vi "Write N LEDs.vi"(7 "Refresh? (T)":bool=TRUE, 8 "Error In":errorcluster, 9 "Colors":u32[](array[colorbox]), 10 "LED Index":u16, 11 "LINX Ref":T1={"IO"=enum."Remote", "Interface"=enum."Serial", "LINX Device Config"={"Interface"=enum."Serial", "COM Port"="COM13", "TCP Configuration"={"IP Address"="", "Port"=0}, "Device Family"=1, "Device ID"=1, "Device Name"="myRIO-1900", "TCP Ref"=refnum, "Channels"={"DI"=[0, 1, 2, 3, 4, 5, 6, 7, 8, 9, 10, 11, 12, 13, 14, 15, 16, 17, 18, 19, 20, 21, 22, 23, 24, 25, 26, 27, 28, 29, 30, 31, 32, 33, 34, 35, 36, 37, 38, 39, 40, 41, 42, 43, 44, 45, 46], "DO"=[0, 1, 2, 3, 4, 5, 6, 7, 8, 9, 10, 11, 12, 13, 14, 15, 16, 17, 18, 19, 20, 21, 22, 23, 24, 25, 26, 27, 28, 29, 30, 31, 32, 33, 34, 35, 36, 37, 38, 39, 40, 41, 42, 43, 44, 45, 46], "AI"=[0, 1, 2, 3, 4, 5, 6, 7, 8, 9, 10, 11], "AO"=[], "PWM"=[3, 5, 6, 9, 10], "QE"=[], "UART"=[0, 1], "I2C 2"=[0], "SPI"=[0], "CAN"=[], "Servo"=[], "AI Ref (V)"=0.0, "AI Resolution (Bits)"=0, "AO Ref (V)"=0.0, "AO Resolution (Bits)"=0}}}) -> (0 "Error Out":errorcluster, 3 "LINX Ref":T1={"IO"=enum."Remote", "Interface"=enum."Serial", "LINX Device Config"={"Interface"=enum."Serial", "COM Port"="COM13", "TCP Configuration"={"IP Address"="", "Port"=0}, "Device Family"=1, "Device ID"=1, "Device Name"="myRIO-1900", "TCP Ref"=refnum, "Channels"={"DI"=[0, 1, 2, 3, 4, 5, 6, 7, 8, 9, 10, 11, 12, 13, 14, 15, 16, 17, 18, 19, 20, 21, 22, 23, 24, 25, 26, 27, 28, 29, 30, 31, 32, 33, 34, 35, 36, 37, 38, 39, 40, 41, 42, 43, 44, 45, 46], "DO"=[0, 1, 2, 3, 4, 5, 6, 7, 8, 9, 10, 11, 12, 13, 14, 15, 16, 17, 18, 19, 20, 21, 22, 23, 24, 25, 26, 27, 28, 29, 30, 31, 32, 33, 34, 35, 36, 37, 38, 39, 40, 41, 42, 43, 44, 45, 46], "AI"=[0, 1, 2, 3, 4, 5, 6, 7, 8, 9, 10, 11], "AO"=[], "PWM"=[3, 5, 6, 9, 10], "QE"=[], "UART"=[0, 1], "I2C 2"=[0], "SPI"=[0], "CAN"=[], "Servo"=[], "AI Ref (V)"=0.0, "AI Resolution (Bits)"=0, "AO Ref (V)"=0.0, "AO Resolution (Bits)"=0}}})   [LabVIEW 2020, in "LMH-LINX.lvlib" / "WS2812.lvlib"]
doc: "Set the R, G, B color of N LEDs starting at the user specififed LED index. If Refresh is true (default) the new colors are immediatly displayed. If Refresh is false the new colors are stored in memory but the LEDs are not updated until Refresh is called."
uses:
  WS2812.lvlib
  Private/Type Defs/LINX Ref.ctl
  Private/Type Defs/Platform.ctl
  Private/Type Defs/Interface.ctl
  Private/Device/Type Defs/LINX Device Config.ctl
  Private/Device/Type Defs/TCP Config.ctl
  Private/Device/Type Defs/Channels.ctl
  Private/Type Defs/Error Type.ctl
  LMH-LINX.lvlib
  Private/Device/Device.lvlib
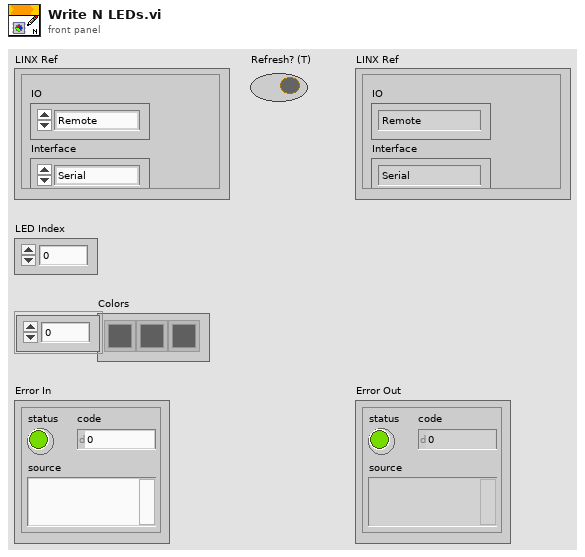
[diagram p1: front panel]
types:
  T1 = typedef "LMH-LINX.lvlib/LINX Ref.ctl" = cluster{"IO":T2, "Interface":T3, "LINX Device Config":T4}
  T2 = typedef "LMH-LINX.lvlib/Platform.ctl" = enum16{"Remote", "Local"}
  T3 = typedef "LMH-LINX.lvlib/Interface.ctl" = enum16{"Serial", "TCP"}
  T4 = typedef "Device.lvlib/LINX Device Config.ctl" = cluster{"Interface":T3, "COM Port":refnum<visa-resource-name>, "TCP Configuration":T5, "Device Family":u8, "Device ID":u8, "Device Name":string, "TCP Ref":refnum<k5>, "Channels":T6}
  T5 = typedef "Device.lvlib/TCP Config.ctl" = cluster{"IP Address":string, "Port":u16}
  T6 = typedef "LMH-LINX.lvlib/Channels.ctl" = cluster{"DI":u8[], "DO":u8[], "AI":u8[], "AO":u8[], "PWM":u8[], "QE":u8[], "UART":u8[], "I2C 2":u8[], "SPI":u8[], "CAN":u8[], "Servo":u8[], "AI Ref (V)":dbl, "AI Resolution (Bits)":u8, "AO Ref (V)":dbl, "AO Resolution (Bits)":u8}
  T7 = typedef "LMH-LINX.lvlib/Error Type.ctl" = enum16{"Unknown", "Timeout", "Corrupt Return Packet", "Unable To Connect", "Command Not Supported", "Channel DNE", "Invalid COM Config", "Firmware Version Mismatch", "myRIO Support", "CMD Specific Error", "Local IO Not Supported"}
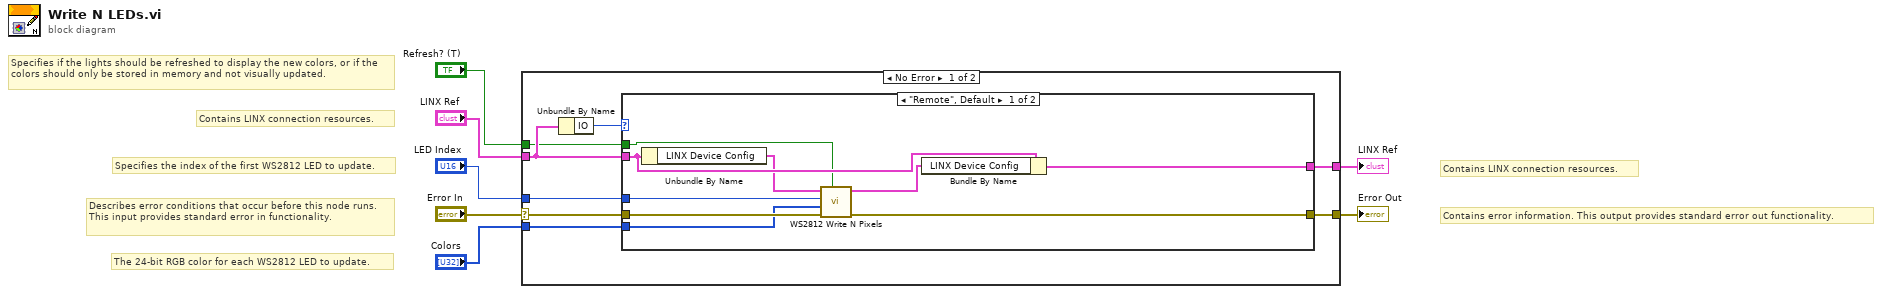
[diagram p0: block diagram]
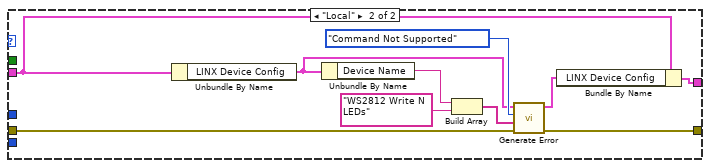
[diagram p2: hidden frame]
diagram:
  # "Specifies if the lights should be refreshed to display the new colors, or if the colors should only be stored in memory and not visually updated."
  # "Specifies the index of the first WS2812 LED to update."
  # "The 24-bit RGB color for each WS2812 LED to update."
  # "Contains LINX connection resources."
  # "Contains error information. This output provides standard error out functionality."
  # "Contains LINX connection resources."
  # "Describes error conditions that occur before this node runs. This input provides standard error in functionality."
  n1 = case shown="No Error" "Error In" {
    selector: "Error In" -> [w14 w35]
    tunnel: "LINX Ref" -> [w13 w36]
    tunnel: [w12 w35] -> w5
    tunnel: [w11 w36] -> w4
    tunnel: "LED Index" -> [w10 _]
    tunnel: "Colors" -> [w9 _]
    tunnel: "Refresh? (T)" -> [w8 _]
    frame No Error {
      n2 = Unbundle By Name(w13) -> ("IO"=w15:T2)
      n3 = case shown="\"Remote\", Default" w15 {
        tunnel: w14 -> [w21 w28]
        tunnel: w13 -> [w24 w25]
        tunnel: [w22 w27] -> w12
        tunnel: [w23 w26] -> w11
        tunnel: w10 -> [w17 _]
        tunnel: w9 -> [w16 _]
        tunnel: w8 -> [w18 _]
        frame "Remote", Default {
          n4 = Unbundle By Name(w24) -> ("LINX Device Config"=w20:T4)
          n5 = call "WS2812 Write N Pixels.vi"("Refresh?"=w18, "Error In"=w21, "Colors"=w16, "Start Pixel Index"=w17, "LINX Device Config"=w20) -> ("Error Out"=w22:errorcluster, "LINX Device Config"=w19:T4)  [unwired: 5 in]
          n6 = Bundle By Name(cluster=w24, "LINX Device Config"=w19) -> (w23:T1)
        }
        frame "Local" {
          n7 = Unbundle By Name(w25) -> ("LINX Device Config"=w30:T4)
          n8 = Unbundle By Name(w30) -> ("Device Name"=w34:string)
          n9 = Build Array(w34, "WS2812 Write N LEDs") -> (w31:string[])
          n10 = call "Generate Error.vi"("Error In"=w28, "Arguments"=w31, "Error Type"=Error_Type."Command Not Supported", "LINX Device Config"=w30) -> ("Error Out"=w27:errorcluster, "Dup LINX Device Config"=w29:T4)  [unwired: 6 in]
          n11 = Bundle By Name(cluster=w25, "LINX Device Config"=w29) -> (w26:T1)
        }
      }
    }
    frame Error {
    }
  }
  "Error Out" <- w5
  "LINX Ref" <- w4
